vi "Calculate Charging Efficiency.vi"(8 "error in":errorcluster, 11 "Particles in":refnum<class "Particle Properties.lvclass">) -> (0 "error out":errorcluster, 2 "f":dbl, 3 "Particles out":refnum<class "Particle Properties.lvclass">)   [LabVIEW 2014, in "Particle Properties.lvclass"]
uses:
  Particle Properties.lvclass
  Particle Properties.lvclass/Particle Properties.ctl
  Atmospheric/Gas Properties/Gas Properties.lvclass/Gas Properties.ctl
  Accessors/Read # of charges.vi
  Accessors/Read Gas Ref.vi
  Accessors/Read D.vi
  Atmospheric/Gas Properties/Accessors/Read T (K).vi
  Atmospheric/Atmospheric Constants.vi
  Atmospheric/Gas Properties/Gas Properties.lvclass
  Atmospheric/Atmospheric Library.lvlib
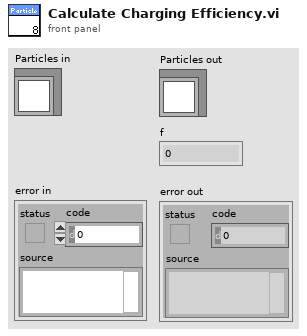
[diagram p1: front panel]
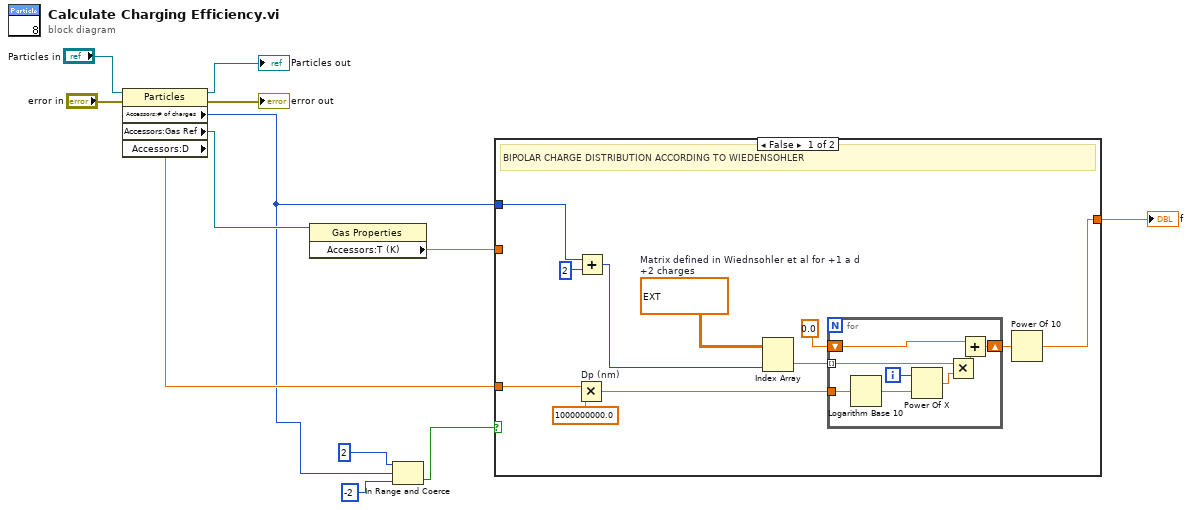
[diagram p0: block diagram]
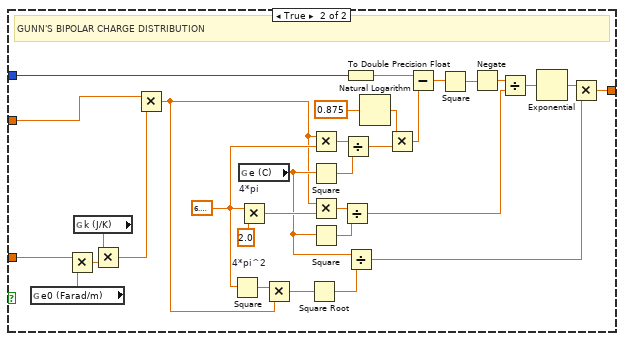
[diagram p2: hidden frame]
diagram:
  n1 = property class="Particles"(reference="Particles in", error in="error in") -> (reference out=→"Particles out":refnum<class "Particle Properties.lvclass">, error out=→"error out":errorcluster, "Accessors:# of charges"=w3:i32, "Accessors:Gas Ref"=w10:refnum<data-value>, "Accessors:D"=w8:dbl)
  n2 = property class="Gas Properties"(reference=w10) -> ("Accessors:T (K)"=w9:dbl)  [unwired: 1 in, 2 out]
  n3 = In Range and Coerce(upper limit=2 ("y"), x=w3, lower limit=-2 ("y")) -> (In Range?=w1:bool)  [unwired: 1 out]
  n4 = case shown="False" w1 {
    tunnel: w8 -> [w13 w61]
    tunnel: w3 -> [w23 w36]
    tunnel: [w16 w41] -> w12
    tunnel: w9 -> [_ w32]
    frame False {
      w15 = ext[][] [[-26.3328, -2.3197, -0.0003, -2.3484, -44.475599999999999998], [35.9044, 0.6175, -0.1014, 0.6044, 79.3772], [-21.4608, 0.6201, 0.3073, 0.48, -62.89], [7.0867, -0.110500000000000000003, -0.3372, 0.00130000000000000000004, 26.4492], [-1.30880000000000000005, -0.125999999999999999994, 0.102300000000000000003, -0.1553, -5.748], [0.1051, 0.0297, -0.0105, 0.031999999999999999999, 0.5049]]  # Matrix defined in Wiednsohler et al for +1 a d +2 charges
      # "BIPOLAR CHARGE DISTRIBUTION ACCORDING TO WIEDENSOHLER"
      n5 = Multiply "Dp (nm)"(x=w13, y=1000000000.0) -> (x*y=w21:dbl)
      n6 = Add(x=w23, y=2) -> (x+y=w20:i32)
      n7 = Index Array(array=w15, index (col)=w20) -> (element=w19:ext[])  [unwired: 1 in]
      n8 = for {
        tunnel: w21 -> [w31]
        tunnel: w19 -> [w27] mode=indexing
        shift-right: [w26] -> w17
        shift-left: 0.0 -> [w24]
        i -> [w29]
        n9 = Logarithm Base 10(1:w31) -> (0:w30:dbl)
        n10 = Power Of X(1:w30, 2:w29) -> (0:w28:dbl)
        n11 = Multiply(x=w27, y=w28) -> (x*y=w25:ext)
        n12 = Add(x=w24, y=w25) -> (x+y=w26:ext)
      }
      n13 = Power Of 10(x=w17) -> (10^x=w16:ext)
    }
    frame True {
      w39 = 6.283185307179586
      # "GUNN'S BIPOLAR CHARGE DISTRIBUTION"
      n14 = global read "Atmospheric Constants.vi" "e0 (Farad/m)"() -> (w59:dbl)
      n15 = Multiply(x=w61, y=w59) -> (x*y=w63:dbl)
      n16 = global read "Atmospheric Constants.vi" "k (J/K)"() -> (w60:dbl)
      n17 = Multiply(x=w60, y=w63) -> (x*y=w62:dbl)
      n18 = Multiply ("Dp*T*k*e0")(x=w32, y=w62) -> (x*y=w37:dbl)
      n19 = Square "4*pi^2"(x=w39) -> (x^2=w38:dbl)
      n20 = global read "Atmospheric Constants.vi" "e (C)"() -> (w40:dbl)
      n21 = Multiply "4*pi"(x=w39, y=2.0) -> (x*y=w48:dbl)
      n22 = Multiply(x=w38, y=w37) -> (x*y=w58:dbl)
      n23 = Square Root(x=w58) -> (sqrt(x)=w42:dbl)
      n24 = Multiply(x=w37, y=w39) -> (x*y=w57:dbl)
      n25 = Square(x=w40) -> (x^2=w56:dbl)
      n26 = Multiply(x=w37, y=w48) -> (x*y=w47:dbl)
      n27 = Square(x=w40) -> (x^2=w46:dbl)
      n28 = Divide(x=w47, y=w46) -> (x/y=w43:dbl)
      n29 = Divide(x=w57, y=w56) -> (x/y=w55:dbl)
      n30 = To Double Precision Float(number=w36) -> (double precision float=w35:dbl)
      n31 = Divide(x=w40, y=w42) -> (x/y=w33:dbl)
      n32 = Natural Logarithm(1:0.875 ("x")) -> (0:w53:dbl)
      n33 = Multiply(x=w53, y=w55) -> (x*y=w52:dbl)
      n34 = Subtract(x=w35, y=w52) -> (x-y=w51:dbl)
      n35 = Square(x=w51) -> (x^2=w50:dbl)
      n36 = Negate(x=w50) -> (-x=w44:dbl)
      n37 = Divide(x=w44, y=w43) -> (x/y=w45:dbl)
      n38 = Exponential(1:w45) -> (0:w34:dbl)
      n39 = Multiply(x=w34, y=w33) -> (x*y=w41:dbl)
    }
  }
  "f" <- w12
